vi "Increment Counter.vi"() -> (1 "Count":i32)   [LabVIEW 2021]
doc: "This VI increments a counter and outputs the current number of calls since application strat. It is intended to count loops, but can be used for other applications as well."
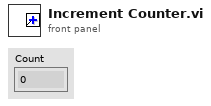
[diagram p1: front panel]
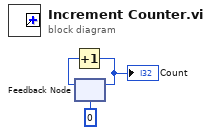
[diagram p0: block diagram]
diagram:
  n1 = feedback #1(0) -> (w2:i32)
  n2 = Increment(x=w2) -> (x+1=w3:i32)
  "Count" <- w3
  n3 = feedback-in #1(w3) -> ()
